vi "K6221_Manage_Monitor.vi"(4 "System Monitor Variables (in)":T2, 5 "Command (in)":T1, 6 "Global Status (in)":T1, 7 "queue (in)":refnum<queue>) -> (0 "System Monitor Variables (out)":T2, 1 "Monitor (out)":T1)   [LabVIEW 2019]
uses:
  Global/Global Variables/System Monitor Cluster.ctl
  K6221/K6221_Cluster.ctl
panel:
  # "K 6221"
  # "K 6221"
  # "K 6221"
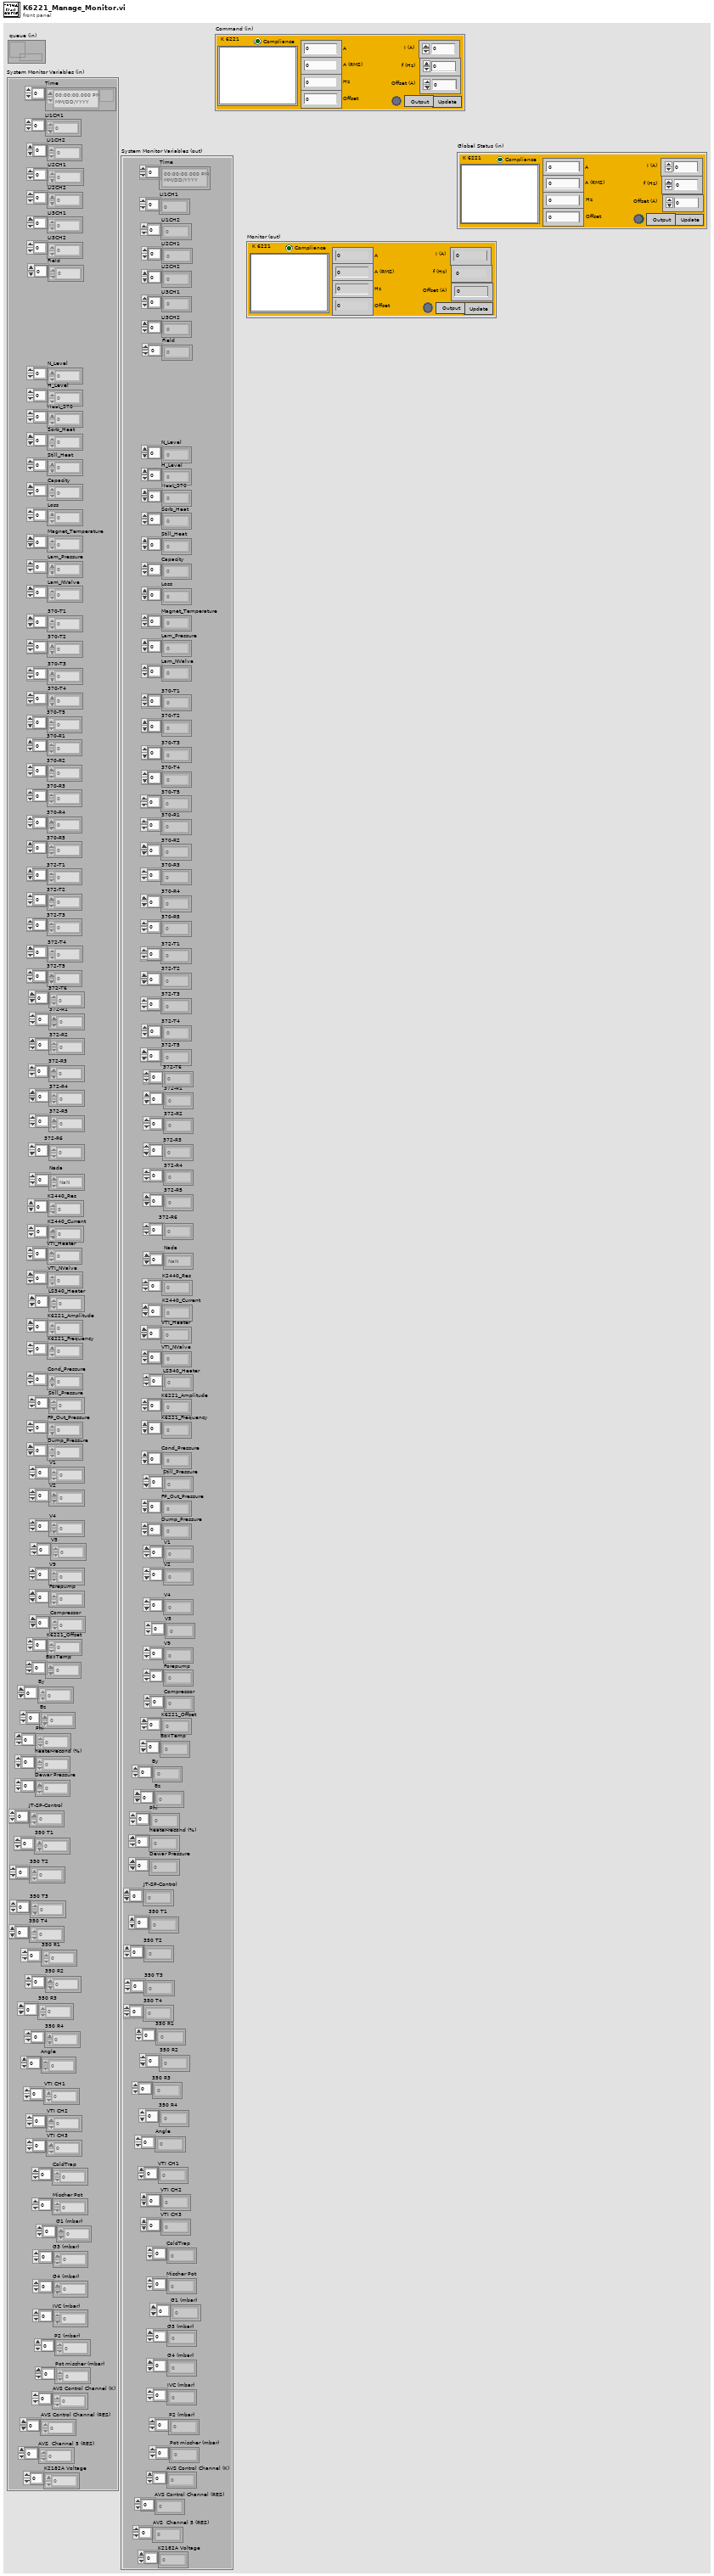
[diagram p1: front panel]
types:
  T1 = typedef "K6221_Cluster.ctl" = cluster{"Plot Window":dbl[][], "A":dbl, "A (RMS)":dbl, "Hz":dbl, "I (A)":dbl, "f (Hz)":dbl, "Update":bool, "Offset":dbl, "Offset (A)":dbl, "Compliance":bool, "Output":bool, "Output Status":bool}
  T2 = typedef "System Monitor Cluster.ctl" = cluster{"Time":timestamp[], "LI1CH1":dbl[], "LI1CH2":dbl[], "LI2CH1":dbl[], "LI2CH2":dbl[], "LI3CH1":dbl[], "LI3CH2":dbl[], "Field":dbl[], "N_Level":dbl[], "H_Level":dbl[], "Heat_370":dbl[], "Sorb_Heat":dbl[], "Still_Heat":dbl[], "Capacity":dbl[], "Loss":dbl[], "Magnet_Temperature":dbl[], "Lam_Pressure":dbl[], "Lam_NValve":dbl[], "370-T1":dbl[], "370-T2":dbl[], "370-T3":dbl[], "370-T4":dbl[], "370-T5":dbl[], "370-R1":dbl[], "370-R2":dbl[], "370-R3":dbl[], "370-R4":dbl[], "370-R5":dbl[], "372-T1":dbl[], "372-T2":dbl[], "372-T3":dbl[], "372-T4":dbl[], "372-T5":dbl[], "372-T6":dbl[], "372-R1":dbl[], "372-R2":dbl[], "372-R3":dbl[], "372-R4":dbl[], "372-R5":dbl[], "372-R6":dbl[], "Nada":dbl[], "K2440_Res":dbl[], "K2440_Current":dbl[], "VTI_Heater":dbl[], "VTI_NValve":dbl[], "LS340_Heater":dbl[], "K6221_Amplitude":dbl[], "K6221_Frequency":dbl[], "Cond_Pressure":dbl[], "Still_Pressure":dbl[], "FP_Out_Pressure":dbl[], "Dump_Pressure":dbl[], "V1":dbl[], "V2":dbl[], "V4":dbl[], "V5":dbl[], "V9":dbl[], "Forepump":dbl[], "Compressor":dbl[], "K6221_Offset":dbl[], "BoxTemp":dbl[], "By":dbl[], "Bz":dbl[], "Phi":dbl[], "heater-recond (%)":dbl[], "Dewar Pressure ":dbl[], "JT-SP-Control":dbl[], "350 T1":dbl[], "350 T2":dbl[], "350 T3":dbl[], "350 T4":dbl[], "350 R1":dbl[], "350 R2":dbl[], "350 R3":dbl[], "350 R4":dbl[], "Angle":dbl[], "VTI CH1":dbl[], "VTI CH2":dbl[], "VTI CH3":dbl[], "ColdTrap":dbl[], "Mischer Pot":dbl[], "G1 (mbar)":dbl[], "G3 (mbar) ":dbl[], "G4 (mbar)":dbl[], "IVC (mbar)":dbl[], "P2 (mbar) ":dbl[], "Pot mischer (mbar)":dbl[], "AVS Control Channel (K)":dbl[], "AVS Control Channel (RES)":dbl[], "AVS  Channel 5 (RES) ":dbl[], "K2182A Voltage":dbl[]}
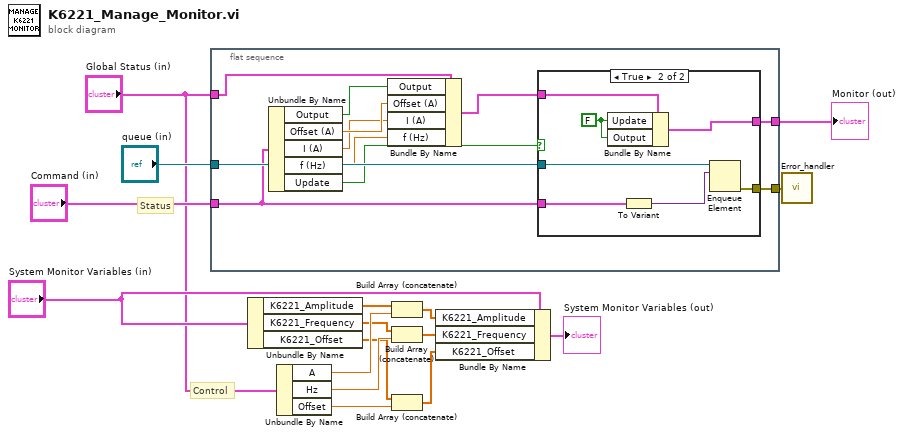
[diagram p0: block diagram]
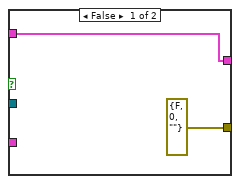
[diagram p2: hidden frame]
diagram:
  # "Status"
  # "Control"
  n1 = flat-sequence {
    tunnel: "queue (in)" -> [w27]
    tunnel: "Command (in)" -> [w25]
    tunnel: [w26] -> w5
    tunnel: "Global Status (in)" -> [w22]
    tunnel: [w23] -> w4
    frame #0 {
      n2 = Unbundle By Name(w25) -> ("Output"=w20:bool, "Offset (A)"=w19:dbl, "I (A)"=w18:dbl, "f (Hz)"=w17:dbl, "Update"=w24:bool)
      n3 = Bundle By Name(cluster=w22, "Output"=w20, "Offset (A)"=w19, "I (A)"=w18, "f (Hz)"=w17) -> (w21:T1)
      n4 = case shown="True" w24 {
        tunnel: w27 -> [_ w36]
        tunnel: w25 -> [_ w33]
        tunnel: [w28 w34] -> w26
        tunnel: w21 -> [w28 w32]
        tunnel: [errorcluster {"status"=FALSE, "code"=0, "source"=""} ("error constant") w31] -> w23
        frame False {
        }
        frame True {
          w30 = FALSE
          n5 = Bundle By Name(cluster=w32, "Update"=w30, "Output"=w30) -> (w34:T1)
          n6 = To Variant(anything=w33) -> (Variant=w35:variant)
          n7 = Enqueue Element(queue=w36, element=w35) -> (error out=w31:errorcluster)  [unwired: 2 in, 2 out]
        }
      }
    }
  }
  n8 = Unbundle By Name("System Monitor Variables (in)") -> ("K6221_Amplitude"=w12:dbl[], "K6221_Frequency"=w10:dbl[], "K6221_Offset"=w2:dbl[])
  n9 = Unbundle By Name("Global Status (in)") -> ("A"=w13:dbl, "Hz"=w9:dbl, "Offset"=w3:dbl)
  n10 = Build Array (concatenate)(w12, w13) -> (w11:dbl[])
  n11 = Build Array (concatenate)(w10, w9) -> (w8:dbl[])
  n12 = Build Array (concatenate)(w2, w3) -> (w1:dbl[])
  n13 = Bundle By Name(cluster="System Monitor Variables (in)", "K6221_Amplitude"=w11, "K6221_Frequency"=w8, "K6221_Offset"=w1) -> (→"System Monitor Variables (out)":T2)
  n14 = call "Error_handler.vi"("error constant"=w4) -> ()
  "Monitor (out)" <- w5
